vi "PortC Controller.vi"(8 "error in":errorcluster) -> ()   [LabVIEW 2015]
doc: "This VI executes continuously carrying out the current operation and responding to updates or new operations. It will often contain the timing or control code that is difficult to place directly in TeleOp. This VI generally opens all sensors and motors and isolates the rest of the robot code from knowing how the operations are carried out."
uses:
  PortC Setpoints.ctl
  PortC Operations.ctl
  Framework/Motor Ref Names Type Def.ctl
  Framework/Robot Global Data.vi
panel:
  out "Current\nCmd":string
  # "Tip: It may be helpful to observe inputs and sensor values.\nYou may also want to display tuning or debugging controls."
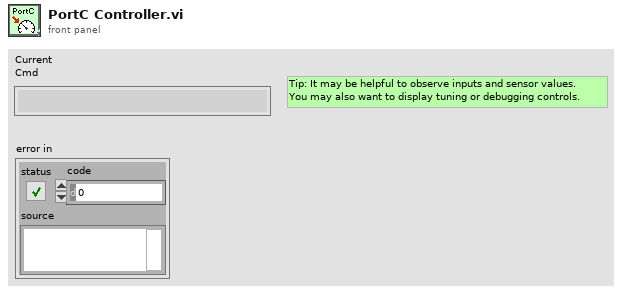
[diagram p1: front panel]
types:
  T1 = typedef "Robot Type Def.ctl" = enum32{"Disabled", "Ghost", "Casper", "Lofty", "Board"}
  T2 = typedef "Motor Ref Names Type Def.ctl" = enum16{"Angular Motor", "Shooter Motor Bottom", "Shooter Motor Top", "Arm Shooter Motor"}
  T3 = typedef "PortC Setpoints.ctl" = cluster{"Operation":T4, "Setpoint":dbl, "Duration":dbl}
  T4 = typedef "PortC Operations.ctl" = enum16{"Reserve", "Read Current", "Immediate", "To Initial Position", "From Initial Position", "Lift Gate"}
  T5 = typedef "Command Status Info.ctl" = cluster{"Name":string, "Status":T6, "notifier out":T7}
  T6 = typedef "Completion Status.ctl" = enum16{"Successful", "Aborted", "Incomplete"}
  T7 = typedef "Completion Notifier.ctl" = refnum<notifier>
  T8 = cluster{"Default Command":T3, "Command Timing":cluster{"Start Time (ms)":u32, "Iterations":i32}, "Command Arguments":cluster{"Command Info":T5, "Description":string, "Default Command":T3, "notifier out":refnum<notifier>, "Subsystem Name":string}}
  T9 = typedef "Addon Motor Type Def.ctl" = cluster{"SwitchDevRef":T10, "LidarRef":T13, "Arm Sensors":cluster{"Front Sensor":T10, "Back Sensor":T10, "Ball Sensor":T10}}
  T10 = typedef "WPI_SwitchDevRef.ctl" = cluster{"DevStatus":errorcluster, "DIO Channel":T11, "CntIndex":T12, "Normally Closed":bool}
  T11 = typedef "FPGA_DIOChannel.ctl" = enum8{"DIO 0", "DIO 1", "DIO 2", "DIO 3", "DIO 4", "DIO 5", "DIO 6", "DIO 7", "DIO 8", "DIO 9", "DIO MXP 0", "DIO MXP 1", "DIO MXP 2", "DIO MXP 3", "DIO MXP 4", "DIO MXP 5", "DIO MXP 6", "DIO MXP 7", "DIO MXP 8", "DIO MXP 9", "DIO MXP 10", "DIO MXP 11", "DIO MXP 12", "DIO MXP 13", "DIO MXP 14", "DIO MXP 15", "Invalid"}
  T12 = typedef "FPGA_CounterCtrSystemIndex.ctl" = enum8{"Ctr 0", "Ctr 1", "Ctr 2", "Ctr 3", "Ctr 4", "Ctr 5", "Ctr 6", "Ctr 7", "Invalid"}
  T13 = typedef "Lidar Type Def.ctl" = cluster{"I2CDevRef":T14}
  T14 = typedef "WPI_I2CDevRef.ctl" = cluster{"DevStatus":errorcluster, "Device Address":u8, "Handle":i32, "I2C Bus":T15}
  T15 = typedef "i2c_bus.ctl" = enum16{"I2C On-Board", "I2C MXP", "Invalid"}
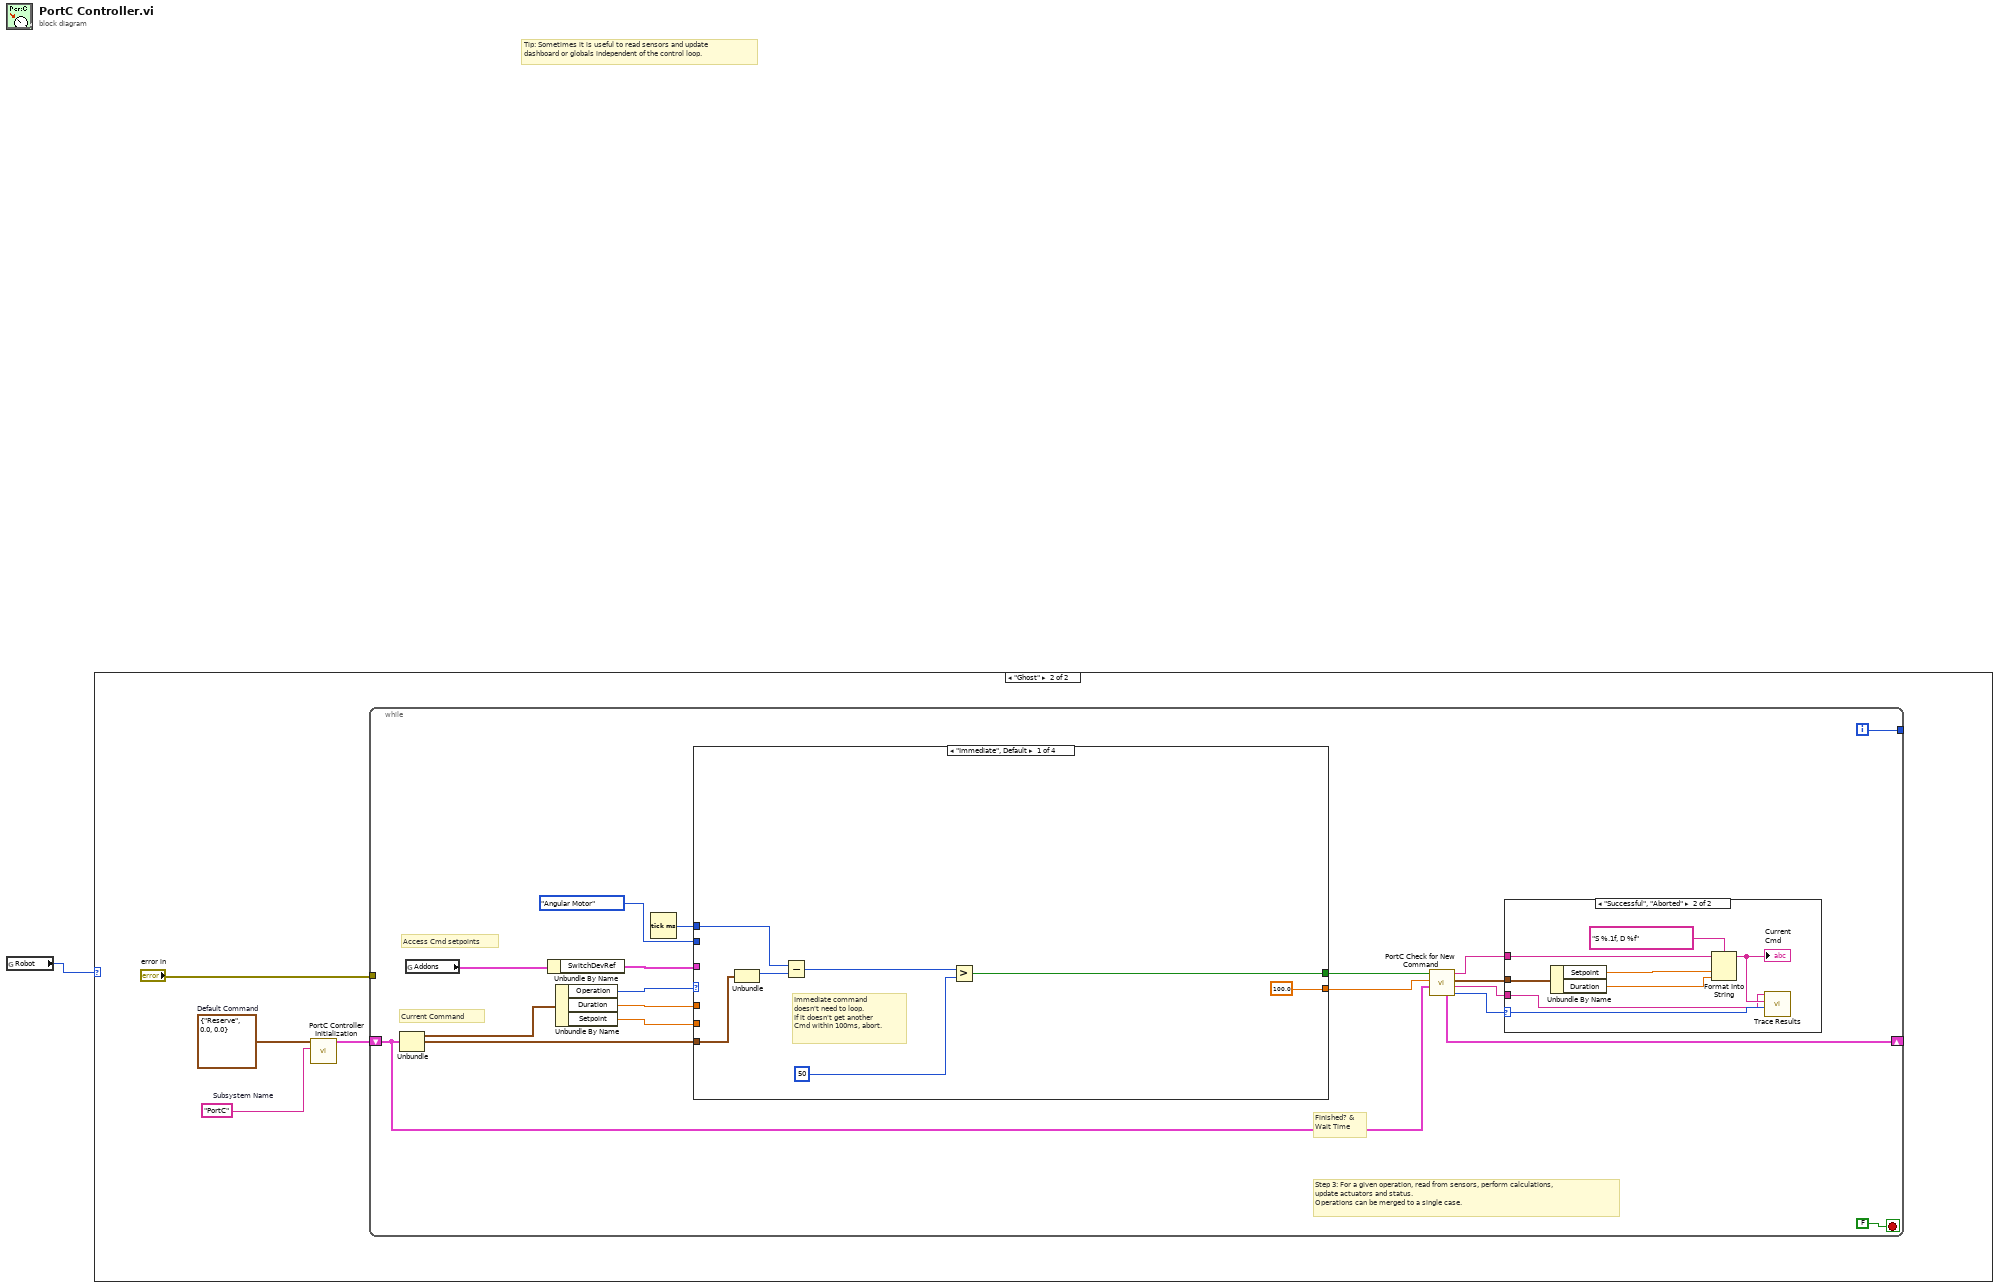
[diagram p0: block diagram]
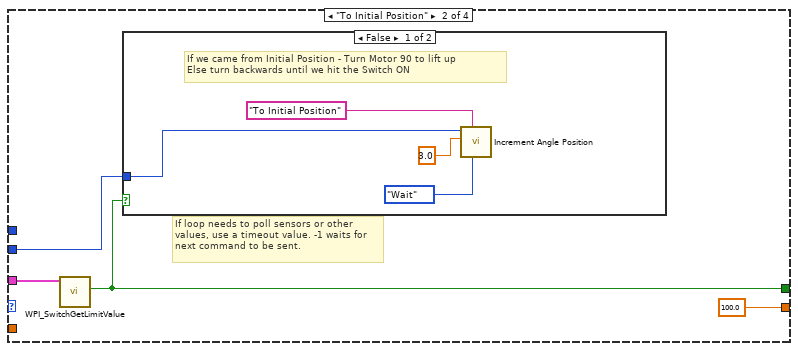
[diagram p4: hidden frame]
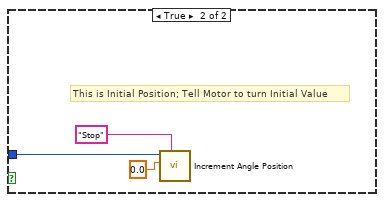
[diagram p5: hidden frame]
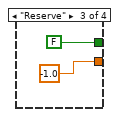
[diagram p6: hidden frame]
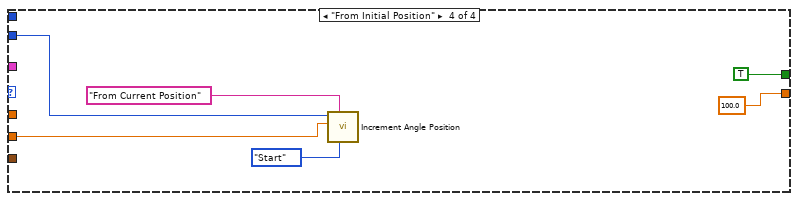
[diagram p7: hidden frame]
diagram:
  # "Tip: Sometimes it is useful to read sensors and update\ndashboard or globals independent of the control loop."
  n1 = global read "Robot Global Data.vi" "Robot"() -> (w1:T1)
  n2 = case shown="\"Ghost\"" w1 {
    frame Default {
    }
    frame "Ghost" {
      w2 = T3 {"Operation"=enum."Reserve", "Setpoint"=0.0, "Duration"=0.0}  # Default Command
      w3 = "PortC"  # Subsystem Name
      n3 = call "PortC Controller Initialization.vi"("Subsystem Name"=w3, "Default Command"=w2) -> ("Command Info"=w4:T8)  [unwired: 9 in]
      n4 = while {
        shift-right: [w15] -> _
        shift-left: w4 -> [w16]
        tunnel: [w23] -> _
        tunnel: "error in" -> [_]
        i -> [w23]
        stop <- FALSE stop-if-true
        # "Current Command"
        # "Access Cmd setpoints"
        # "Finished? &\nWait Time"
        # "Step 3: For a given operation, read from sensors, perform calculations,\nupdate actuators and status.\nOperations can be merged to a single case."
        n5 = Unbundle(w16) -> ("Default Command"=w22:T3, "Command Timing"=w18:cluster{"Start Time (ms)":u32, "Iterations":i32})  [unwired: 1 out]
        n6 = global read "Robot Global Data.vi" "Addons"() -> (w7:T9)
        n7 = Unbundle By Name(w7) -> ("SwitchDevRef"=w8:T10)
        n8 = Unbundle By Name(w22) -> ("Operation"=w21:T4, "Duration"=w20:dbl, "Setpoint"=w17:dbl)
        n9 = Tick Count (ms)() -> (millisecond timer value=w19:u32)
        n10 = case shown="\"Immediate\", Default" w21 {
          tunnel: [100.0 100.0 -1.0 100.0] -> w13
          tunnel: [w33 w41 FALSE ("ignore previous (F)") TRUE ("ignore previous (F)")] -> w14
          tunnel: w18 -> [w35 _ _ _]
          tunnel: w20 -> [_ _ _ _]
          tunnel: w19 -> [w34 _ _ _]
          tunnel: w17 -> [_ _ _ w53]
          tunnel: w8 -> [_ w42 _ _]
          tunnel: Motor_Ref_Names_Type_Def."Angular Motor" ("Motor Ref Names") -> [_ w40 _ w54]
          frame "Immediate", Default {
            # "Immediate command\ndoesn't need to loop.\nIf it doesn't get another\nCmd within 100ms, abort."
            n11 = Unbundle(w35) -> ("Start Time (ms)"=w38:u32)  [unwired: 1 out]
            n12 = Subtract(x=w34, y=w38) -> (x-y=w37:u32)
            n13 = Greater?(x=w37, y=u8 50 ("Left Motor")) -> (0:w33:bool)
          }
          frame "To Initial Position" {
            # "If loop needs to poll sensors or other\nvalues, use a timeout value. -1 waits for\nnext command to be sent."
            n14 = call <vilib>:"WPI_SwitchGetLimitValue.vi"("SwitchDevRef"=w42) -> ("Switch Pressed"=w41:bool)  [unwired: 8 in, 2 out]
            n15 = case shown="False" w41 {
              tunnel: w40 -> [w44 w48]
              frame False {
                # "If we came from Initial Position - Turn Motor 90 to lift up\nElse turn backwards until we hit the Switch ON"
                n16 = call "Increment Angle Position.vi"("Synchronization"=enum16{"Start", "Wait"}."Wait", "Description"="To Initial Position", "Angle"=3.0, "Motor ID"=w44) -> ()  [unwired: 7 in, 1 out]
              }
              frame True {
                # "This is Initial Position; Tell Motor to turn Initial Value"
                n17 = call "Increment Angle Position.vi"("Description"="Stop", "Angle"=0.0, "Motor ID"=w48) -> ()  [unwired: 8 in, 1 out]
              }
            }
          }
          frame "Reserve" {
          }
          frame "From Initial Position" {
            n18 = call "Increment Angle Position.vi"("Synchronization"=enum16{"Start", "Wait"}."Start", "Description"="From Current Position", "Angle"=w53, "Motor ID"=w54) -> ()  [unwired: 7 in, 1 out]
          }
        }
        n19 = call "PortC Check for New Command.vi"("Current Command"=w16, "Wait time (ms)"=w13, "Finished?"=w14) -> ("Completion"=w9:T6, "Subsystem Name"=w10:string, "Current Command"=w11:T3, "Initial Trace String"=w12:string, "NextCommand"=w15:T8)  [unwired: 4 in]
        n20 = case shown="\"Successful\", \"Aborted\"" w9 {
          selector: w9 -> [_ w32]
          tunnel: w12 -> [_ w28]
          tunnel: w11 -> [_ w29]
          tunnel: w10 -> [_ w25]
          frame "Incomplete", Default {
            # "Continuing current command"
          }
          frame "Successful", "Aborted" {
            # "Report and setup for next command"
            n21 = Unbundle By Name(w29) -> ("Setpoint"=w31:dbl, "Duration"=w26:dbl)
            n22 = Format Into String(format string="S %.1f, D %f", initial string=w28, w31, w26) -> (resulting string=w27:string)  [unwired: 1 in, 1 out]
            "Current\nCmd" <- w27
            n23 = call <vilib>:"Trace Results.vi"("Status of previous command"=w32, "Description"=w27, "Subsystem"=w25) -> ()  [unwired: 9 in]
          }
        }
      }
    }
  }
